vi "Reto(for).vi"() -> ()   [LabVIEW 2020]
panel:
  in  "milliseconds to wait 3":u32=1000
  in  "stop":bool
  out "milliseconds to wait 2":u32=1000
  out "Random":dbl
  out "Iteraciones":i32
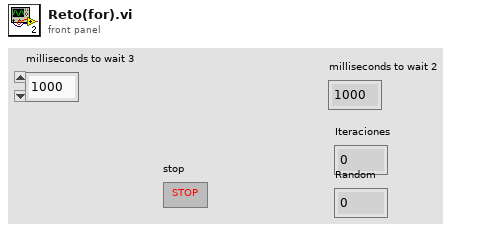
[diagram p1: front panel]
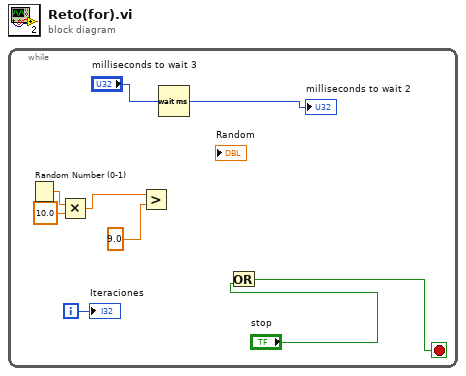
[diagram p0: block diagram]
diagram:
  n1 = while {
    i -> [w7]
    stop <- w4 stop-if-true
    n2 = Random Number (0-1)() -> (number: 0 to 1=w9:dbl)
    n3 = Multiply(x=w9, y=10.0) -> (x*y=w2:dbl)
    n4 = Greater?(x=w2, y=9.0) -> ()  [unwired: 1 out]
    n5 = Wait (ms)(milliseconds to wait="milliseconds to wait 3") -> (millisecond timer value=→"milliseconds to wait 2":u32)
    n6 = Or(y="stop") -> (x .or. y?=w4:bool)  [unwired: 1 in]
    "Iteraciones" <- w7
  }
